vi "Modify Row in Database.vi"(8 "error in (no error)":errorcluster, 10 "Columns (All)":string[](array[string]), 11 "Basic Table in":refnum<class "Basic Table.lvclass">) -> (0 "error out":errorcluster, 3 "Basic Table out":refnum<class "Basic Table.lvclass">)   [LabVIEW 2020, in "Table.lvlib" / "Basic Table.lvclass"]
uses:
  Basic Table.lvclass
  Basic Table.lvclass/Basic Table.ctl
  Table Configuration Interface/Table Configuration Interface.lvclass
  Column Libraries/Column Interface/Column Interface Class/Column Interface.lvclass
  Database Libraries/Database Interfaces/Database Interface Class/Database Interface.lvclass
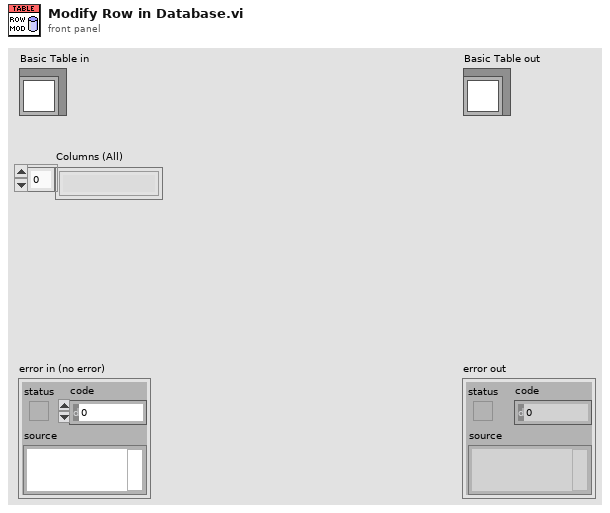
[diagram p1: front panel]
types:
  T1 = map{string, refnum<class "Column Interface.lvclass">}
  T2 = typedef "Database Interfaces.lvlib/Primary Key Info.ctl" = cluster{"Primary Key Column":string, "Display Column":string}
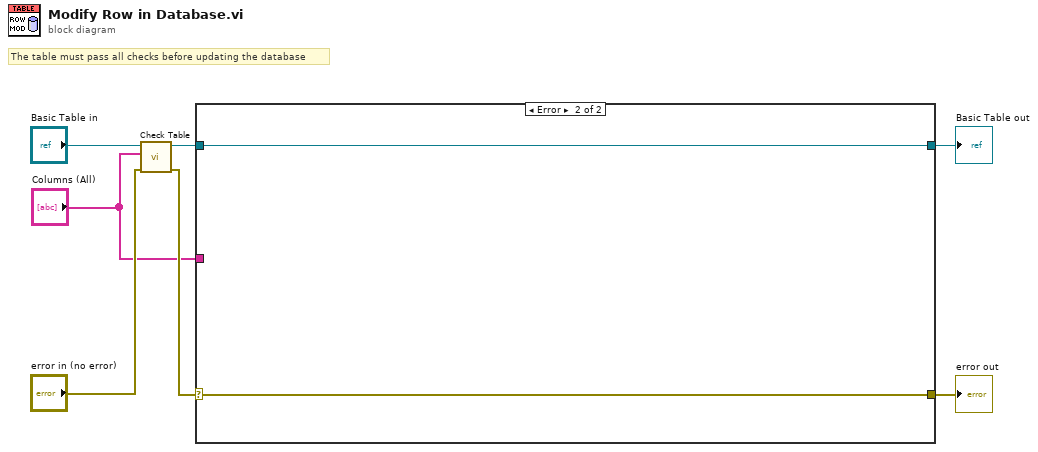
[diagram p0: block diagram]
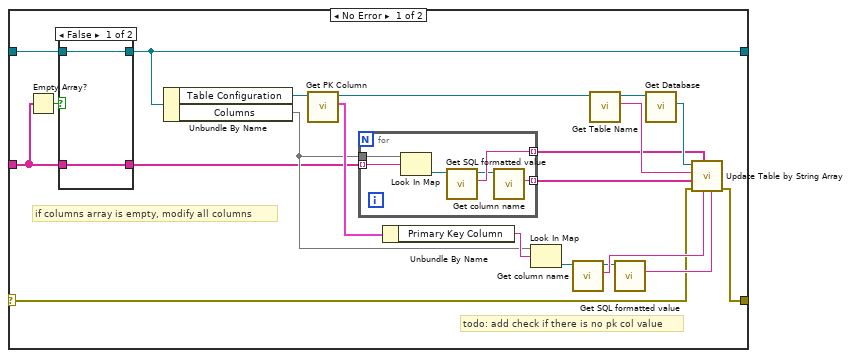
[diagram p2: hidden frame]
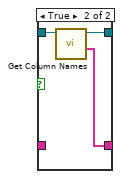
[diagram p3: hidden frame]
diagram:
  # "The table must pass all checks before updating the database"
  n1 = call "Check Table.vi"("error in (no error)"="error in (no error)", "Columns (All)"="Columns (All)", "Table in"="Basic Table in") -> ("error out"=w2:errorcluster, "Table out"=w5:refnum<class "Basic Table.lvclass">)  [unwired: 7 in]
  n2 = case shown="Error" w2 {
    selector: w2 -> [w14 w41]
    tunnel: [w13 w41] -> w7
    tunnel: [w11 w40] -> w6
    tunnel: w5 -> [w12 w40]
    tunnel: "Columns (All)" -> [w9 _]
    frame No Error {
      # "if columns array is empty, modify all columns"
      # "todo: add check if there is no pk col value"
      n3 = Empty Array?(array=w9) -> (empty?=w10:bool)
      n4 = case shown="False" w10 {
        tunnel: w12 -> [w29 w33]
        tunnel: [w29 w32] -> w11
        tunnel: w9 -> [w30 _]
        tunnel: [w30 w31] -> w8
        frame False {
        }
        frame True {
          n5 = call "Get Column Names.vi"("Table in"=w33) -> ("Key Names"=w31:string[], "Table out"=w32:refnum<class "Basic Table.lvclass">)  [unwired: 7 in, 2 out]
        }
      }
      n6 = Unbundle By Name(w11) -> ("Table Configuration"=w23:refnum<class "Table Configuration Interface.lvclass">, "Columns"=w24:T1)
      n7 = call-dynamic "Get PK Column.vi"("Table Configuration Interface in"=w23) -> ("Primary Key"=w26:T2, "Table Configuration Interface out"=w22:refnum<class "Table Configuration Interface.lvclass">)  [unwired: 8 in, 1 out]
      n8 = for {
        tunnel: w8 -> [w39] mode=indexing
        tunnel: w24 -> [w38]
        tunnel: [w36] -> w19 mode=indexing
        tunnel: [w34] -> w20 mode=indexing
        n9 = Look In Map(map=w38, key=w39) -> (value=w37:refnum<class "Column Interface.lvclass">)  [unwired: 1 in, 1 out]
        n10 = call-dynamic "Get SQL formatted value.vi"("Column Interface in"=w37) -> ("Formatted Value"=w36:string, "Column Interface out"=w35:refnum<class "Column Interface.lvclass">)  [unwired: 8 in, 1 out]
        n11 = call-dynamic "Get column name.vi"("Column Interface in"=w35) -> ("Name"=w34:string)  [unwired: 8 in, 2 out]
      }
      n12 = Unbundle By Name(w26) -> ("Primary Key Column"=w25:string)
      n13 = Look In Map(map=w24, key=w25) -> (value=w16:refnum<class "Column Interface.lvclass">)  [unwired: 1 in, 1 out]
      n14 = call-dynamic "Get column name.vi"("Column Interface in"=w16) -> ("Name"=w17:string, "Column Interface out"=w15:refnum<class "Column Interface.lvclass">)  [unwired: 8 in, 1 out]
      n15 = call-dynamic "Get Table Name.vi"("Table Configuration Interface in"=w22) -> ("Table Name"=w21:string, "Table Configuration Interface out"=w28:refnum<class "Table Configuration Interface.lvclass">)  [unwired: 8 in, 1 out]
      n16 = call-dynamic "Get SQL formatted value.vi"("Column Interface in"=w15) -> ("Formatted Value"=w18:string)  [unwired: 8 in, 2 out]
      n17 = call-dynamic "Get Database.vi"("Table Configuration Interface in"=w28) -> ("Database"=w27:refnum<class "Database Interface.lvclass">)  [unwired: 8 in, 2 out]
      n18 = call-dynamic "Update Table by String Array.vi"("PK value"=w18, "PK column"=w17, "data"=w19, "error in (no error)"=w14, "columns"=w20, "table"=w21, "Database Interface in"=w27) -> ("error out"=w13:errorcluster)  [unwired: 3 in, 1 out]
    }
    frame Error {
    }
  }
  "error out" <- w7
  "Basic Table out" <- w6
